vi "VariablesLocal.vi"() -> ()   [LabVIEW 2020]
panel:
  out "String":string
  out "initialized array":dbl[](array[numeric])
  in  "Thermometer":dbl(slide) scale=0.0..100.0
  out "Boolean 2":bool
  in  "Boolean":bool
  in  "stop":bool
  out "Numeric 3":i32
  out "Numeric 2":i32
  out "Numeric":i32
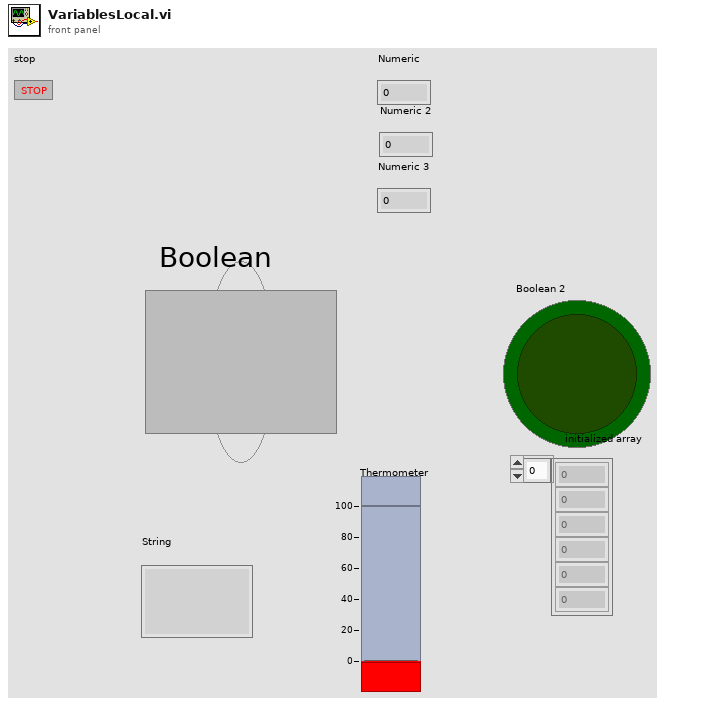
[diagram p1: front panel]
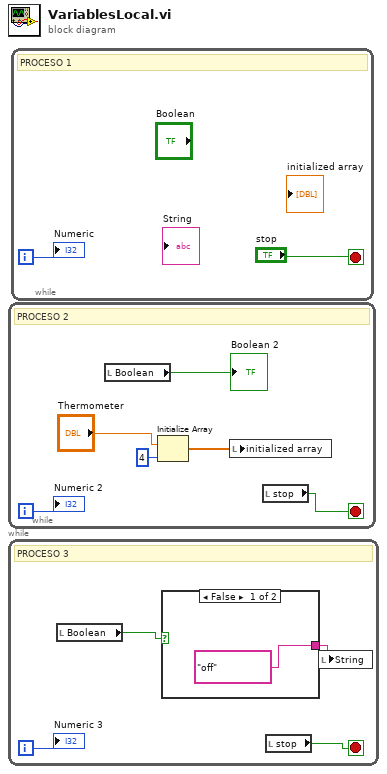
[diagram p0: block diagram]
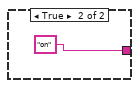
[diagram p2: hidden frame]
diagram:
  n1 = while {
    i -> [w5]
    stop <- w6 stop-if-true
    # "PROCESO 2"
    n2 = local read "Boolean"() -> (→"Boolean 2":bool)
    n3 = Initialize Array("Thermometer", 4 ("dimension size")) -> (w1:dbl[])
    n4 = local write "initialized array"(w1) -> ()
    n5 = local read "stop"() -> (w6:bool)
    "Numeric 2" <- w5
  }
  n6 = while {
    i -> [w9]
    stop <- w10 stop-if-true
    # "PROCESO 3"
    n7 = local read "Boolean"() -> (w8:bool)
    n8 = case shown="False" w8 {
      tunnel: ["off" "on"] -> w7
      frame False {
      }
      frame True {
      }
    }
    n9 = local read "stop"() -> (w10:bool)
    n10 = local write "String"(w7) -> ()
    "Numeric 3" <- w9
  }
  n11 = while {
    i -> [w14]
    stop <- "stop" stop-if-true
    # "PROCESO 1"
    "Numeric" <- w14
  }
